vi "HandleError.vi"(7 "code":i32) -> (5 "out_message":string)   [LabVIEW 2026]
uses:
  vision_core_c/bin/error_messages.dll
  <vilib>/Utility/error.llb/Trim Whitespace (string).vi
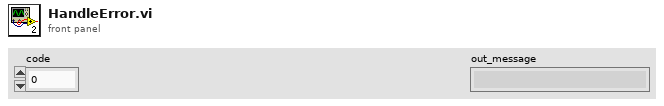
[diagram p1: front panel]
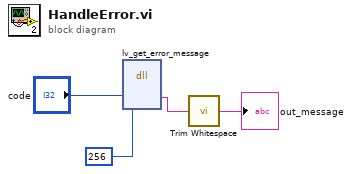
[diagram p0: block diagram]
diagram:
  n1 = dll-call lib="D:/git_proj/LabC-Vision/vision_core_c/bin/error_messages.dll" fn="lv_get_error_message"("code"="code", "out_message_size"=256) -> ("out_message"=w2:string)  [unwired: 7 in, 2 out]
  n2 = call-poly <vilib>:"Trim Whitespace.vi"("string"=w2) -> ("trimmed string"=→"out_message":string)  [unwired: 1 in]
